vi "Timer Module teardown.vi"(8 "error in (no error)":errorcluster, 11 "Module ID":i32) -> (0 "error out":errorcluster)   [LabVIEW 2018]
doc: "_____\nCreated using Delacor QMH Event Scripter 4.1.0.76."
uses:
  Libraries/Timer Module/Timer Module.lvlib
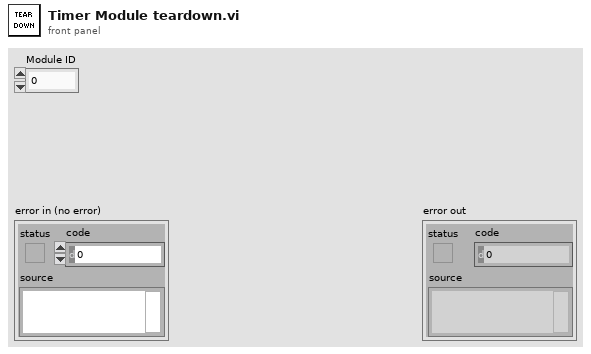
[diagram p1: front panel]
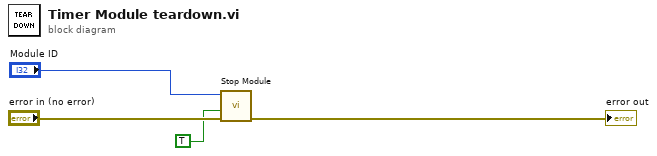
[diagram p0: block diagram]
diagram:
  n1 = call "Stop Module.vi"("error in (no error)"="error in (no error)", "Wait for Module to stop? (F)"=TRUE, "Module ID"="Module ID") -> ("error out"=→"error out":errorcluster)  [unwired: 8 in]
